vi "Kill_Matlab_Script.vi"() -> ()   [LabVIEW 2022 SP3]
panel:
  out "standard output 2":string
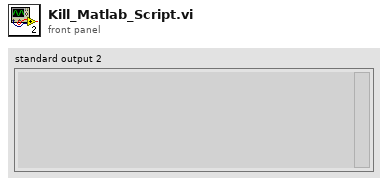
[diagram p1: front panel]
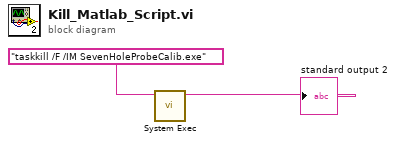
[diagram p0: block diagram]
diagram:
  n1 = call <vilib>:"System Exec.vi"("command line"="taskkill /F /IM SevenHoleProbeCalib.exe") -> ("standard output"=→"standard output 2":string)  [unwired: 7 in, 3 out]
